vi "FTW-Request-Deserialize.vi"(0 "Message":string, 11 "error in":errorcluster) -> (4 "Message Header":string, 6 "Message Body":string, 15 "error out":errorcluster)   [LabVIEW 2013, in "FTW-Actor.lvlib" / "FTW-Request.lvclass"]
uses:
  FTW-Request.lvclass
  Core/src/Reflection/FTW-Reflection-Type.vi
  Core/src/JSON/FTW-JSON-Core-LibraryFilepath.vi
  Core/src/JSON/FTW-JSON-Core-GetFlattenedValue.vi
  Core/src/JSON/FTW-JSON-Core-LibraryError.vi
  Core/utils/CodeGen/JSON Deserialize/FTW-JSON-Deserialize.xnode
panel:
  # "Inputs"
  # "Outputs"
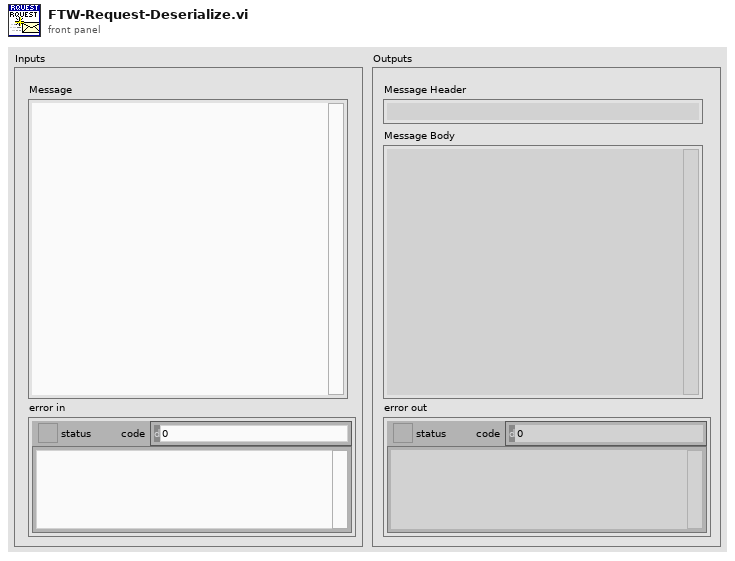
[diagram p1: front panel]
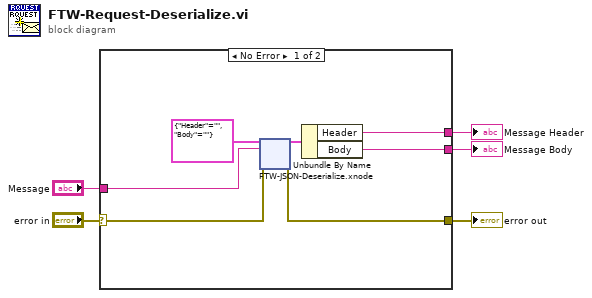
[diagram p0: block diagram]
diagram:
  n1 = case shown="No Error" "error in" {
    selector: "error in" -> [w11 w47]
    tunnel: [w10 w47] -> w5
    tunnel: "Message" -> [w12 _]
    tunnel: [w7 _] -> w2
    tunnel: [w6 _] -> w1
    frame No Error {
      n2 = xnode "FTW-JSON-Deserialize.xnode"("Type and Defaults"=cluster{"Header":string, "Body":string} {"Header"="", "Body"=""}, "JSON String"=w12, "error in"=w11) -> ("Values"=w8:cluster{"Header":string, "Body":string}, "error out"=w10:errorcluster)
      n3 = Unbundle By Name(w8) -> ("Header"=w7:string, "Body"=w6:string)
    }
    frame Error {
    }
  }
  "error out" <- w5
  "Message Header" <- w2
  "Message Body" <- w1
